vi "Connect.vi"(8 "error in (no error)":errorcluster, 10 "Y-Axis VISA Resource Name":refnum<visa-resource-name>, 11 "Z-Axis VISA Resource Name":refnum<visa-resource-name>) -> (0 "error out":errorcluster, 2 "Y-Axis VISA Resource Name Out":refnum<visa-resource-name>, 3 "Z-Axis VISA Resource Name Out":refnum<visa-resource-name>)   [LabVIEW 2019]
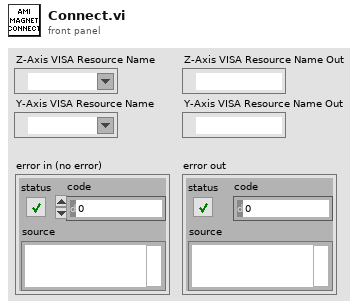
[diagram p1: front panel]
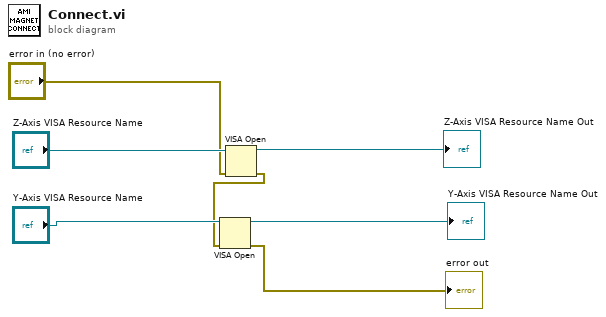
[diagram p0: block diagram]
diagram:
  n1 = VISA Open(error in (no error)="error in (no error)", VISA resource name="Z-Axis VISA Resource Name") -> (VISA resource name=→"Z-Axis VISA Resource Name Out":refnum<visa-resource-name>, error out=w2:errorcluster)  [unwired: 3 in]
  n2 = VISA Open(error in (no error)=w2, VISA resource name="Y-Axis VISA Resource Name") -> (VISA resource name=→"Y-Axis VISA Resource Name Out":refnum<visa-resource-name>, error out=→"error out":errorcluster)  [unwired: 3 in]
